vi "DAQ采集.vi"() -> ()   [LabVIEW 2020]
panel:
  out "data":dbl
  out "波形图":dynamicdata(graph)
  in  "停止":bool
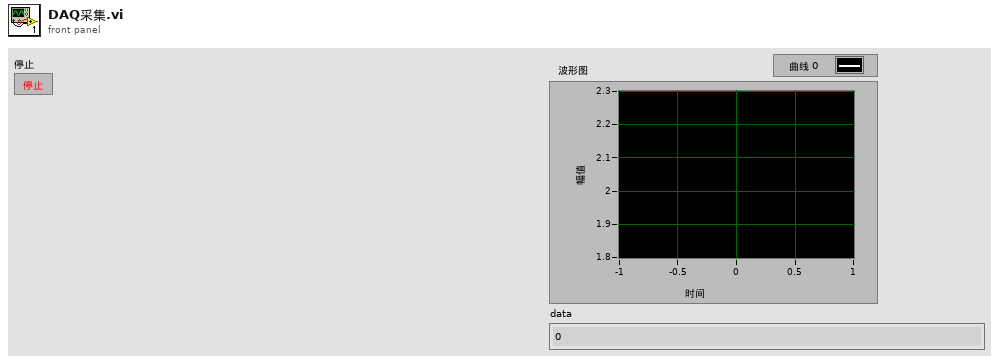
[diagram p1: front panel]
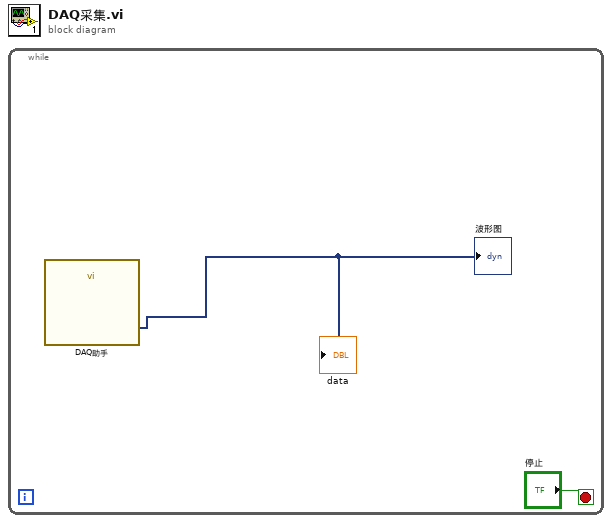
[diagram p0: block diagram]
diagram:
  n1 = while {
    stop <- "停止" stop-if-true
    n2 = call "DAQ助手"() -> ("data"=→"波形图" →"data":dynamicdata)  [unwired: 17 in, 2 out]
  }
